vi "HandleCatch.vi"(8 "error in (no error)":errorcluster, 11 "Toggle?":bool) -> (0 "error out":errorcluster, 3 "ElevatedPassMode":T1)   [LabVIEW 2013]
uses:
  ElevatedPassMode.ctl
panel:
  in  "InitState":T1
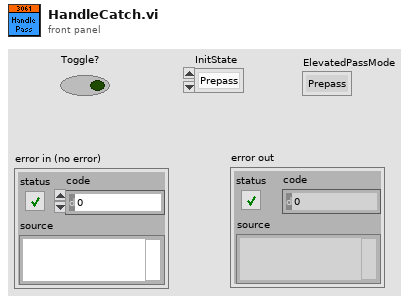
[diagram p1: front panel]
types:
  T1 = typedef "ElevatedPassMode.ctl" = enum16{"Prepass", "Pass", "Stop"}
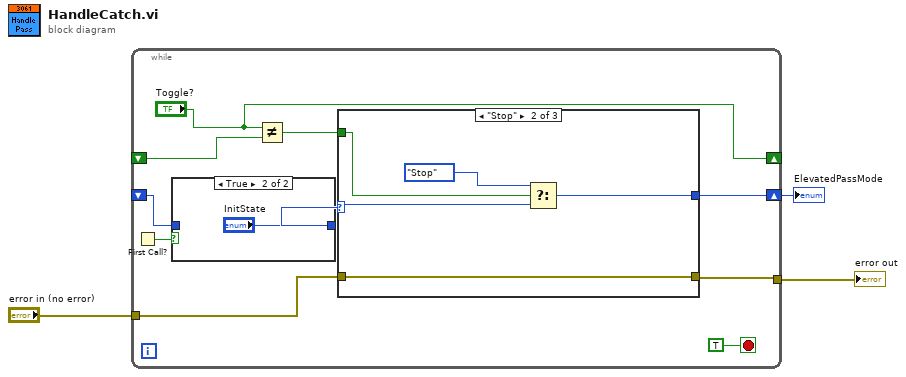
[diagram p0: block diagram]
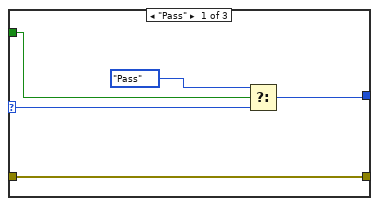
[diagram p3: hidden frame]
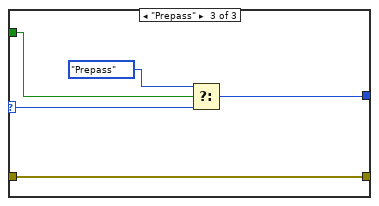
[diagram p4: hidden frame]
diagram:
  n1 = while {
    shift-right: ["Toggle?"] -> _
    shift-left: _ -> [w9]
    tunnel: "error in (no error)" -> [w11]
    tunnel: [w10] -> w2
    shift-right: [w5] -> w1
    shift-left: _ -> [w4]
    stop <- TRUE stop-if-true
    n2 = First Call?() -> (First Call?: T/F=w12:bool)
    n3 = case shown="True" w12 {
      tunnel: [w14 "InitState"] -> w6
      tunnel: w4 -> [w14 _]
      frame False {
      }
      frame True {
      }
    }
    n4 = Not Equal?(x="Toggle?", y=w9) -> (x != y?=w8:bool)
    n5 = case shown="\"Stop\"" w6 {
      selector: w6 -> [w20 w22 w30]
      tunnel: w11 -> [w19 w25 w27]
      tunnel: [w19 w25 w27] -> w10
      tunnel: w8 -> [w18 w24 w29]
      tunnel: [w17 w21 w28] -> w5
      frame "Pass" {
        n6 = Select(t=ElevatedPassMode."Pass" ("ElevatedPassMode"), s=w18, f=w20) -> (s? t:f=w17:T1)
      }
      frame "Stop" {
        n7 = Select(t=ElevatedPassMode."Stop" ("ElevatedPassMode"), s=w24, f=w22) -> (s? t:f=w21:T1)
      }
      frame "Prepass" {
        n8 = Select(t=ElevatedPassMode."Prepass" ("ElevatedPassMode"), s=w29, f=w30) -> (s? t:f=w28:T1)
      }
    }
  }
  "error out" <- w2
  "ElevatedPassMode" <- w1
